vi "PDS_name_generation.vi"(2 "output cluster":T1) -> (4 "Generic Name":string)   [LabVIEW 2023]
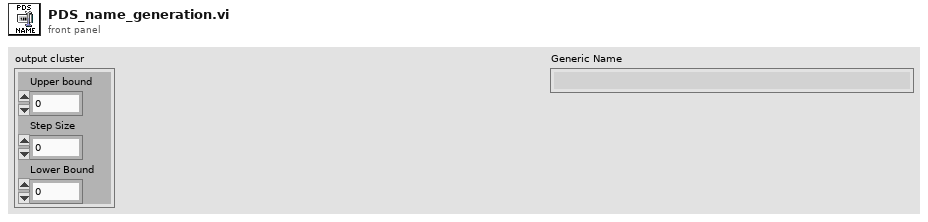
[diagram p1: front panel]
types:
  T1 = cluster{"Upper bound":dbl, "Step Size":dbl, "Lower Bound":dbl}
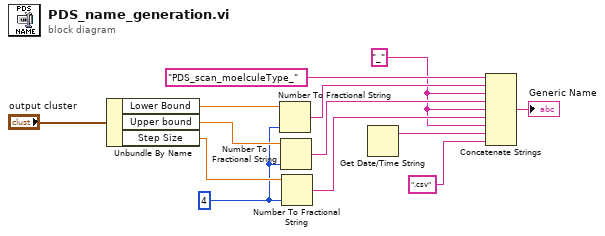
[diagram p0: block diagram]
diagram:
  w4 = "_"
  w9 = i16 4 ("precision (6)")
  n1 = Unbundle By Name("output cluster") -> ("Lower Bound"=w12:dbl, "Upper bound"=w11:dbl, "Step Size"=w10:dbl)
  n2 = Number To Fractional String(number=w12, precision (6)=w9) -> (F-format string=w7:string)  [unwired: 2 in]
  n3 = Number To Fractional String(number=w11, precision (6)=w9) -> (F-format string=w6:string)  [unwired: 2 in]
  n4 = Number To Fractional String(number=w10, precision (6)=w9) -> (F-format string=w5:string)  [unwired: 2 in]
  n5 = Get Date/Time String() -> (date string=w3:string)  [unwired: 3 in, 1 out]
  n6 = Concatenate Strings("PDS_scan_moelculeType_", w7, w4, w6, w4, w5, w4, w3, ".csv") -> (→"Generic Name":string)
